vi "Main_21A.vi"() -> ()   [LabVIEW 2024]
uses:
  Cluster_Start-End Keys.ctl
  Utility/Universal Utility/TypeDefs_Utility/Cluster_Row-Column.ctl
  9e3f57c0-2ef8-4495-8287-c6a42a5fb955.vi
  Utility/Universal Utility/TypeDefs_Utility/ENUM_4 Directions U-D-L-R.ctl
  Utility/Universal Utility/TypeDefs_Utility/ENUM_8 Directions U-D-L-R.ctl
  ENUM_Numeric Keys.ctl
  ENUM_Arrow Keys.ctl
panel:
  out "concatenated string":string
  out "Array":string[](array[string])
  out "Robot 3 to 2":cluster{"Array":cluster{"Array":string[]}[]}[](array[cluster])
  out "2 to 1 Robot":cluster{"Array":string[]}[](array[cluster])
  out "counts":i32[](array[numeric])
  out "Number":i32[](array[numeric])
  in  "Select Data":enum32{"Example", "Puzzle"}(tab)
  in  "Example":string="029A\n980A\n179A\n456A\n379A"
  in  "Puzzle":string="129A\n974A\n805A\n671A\n386A"
  out "Answer":u32
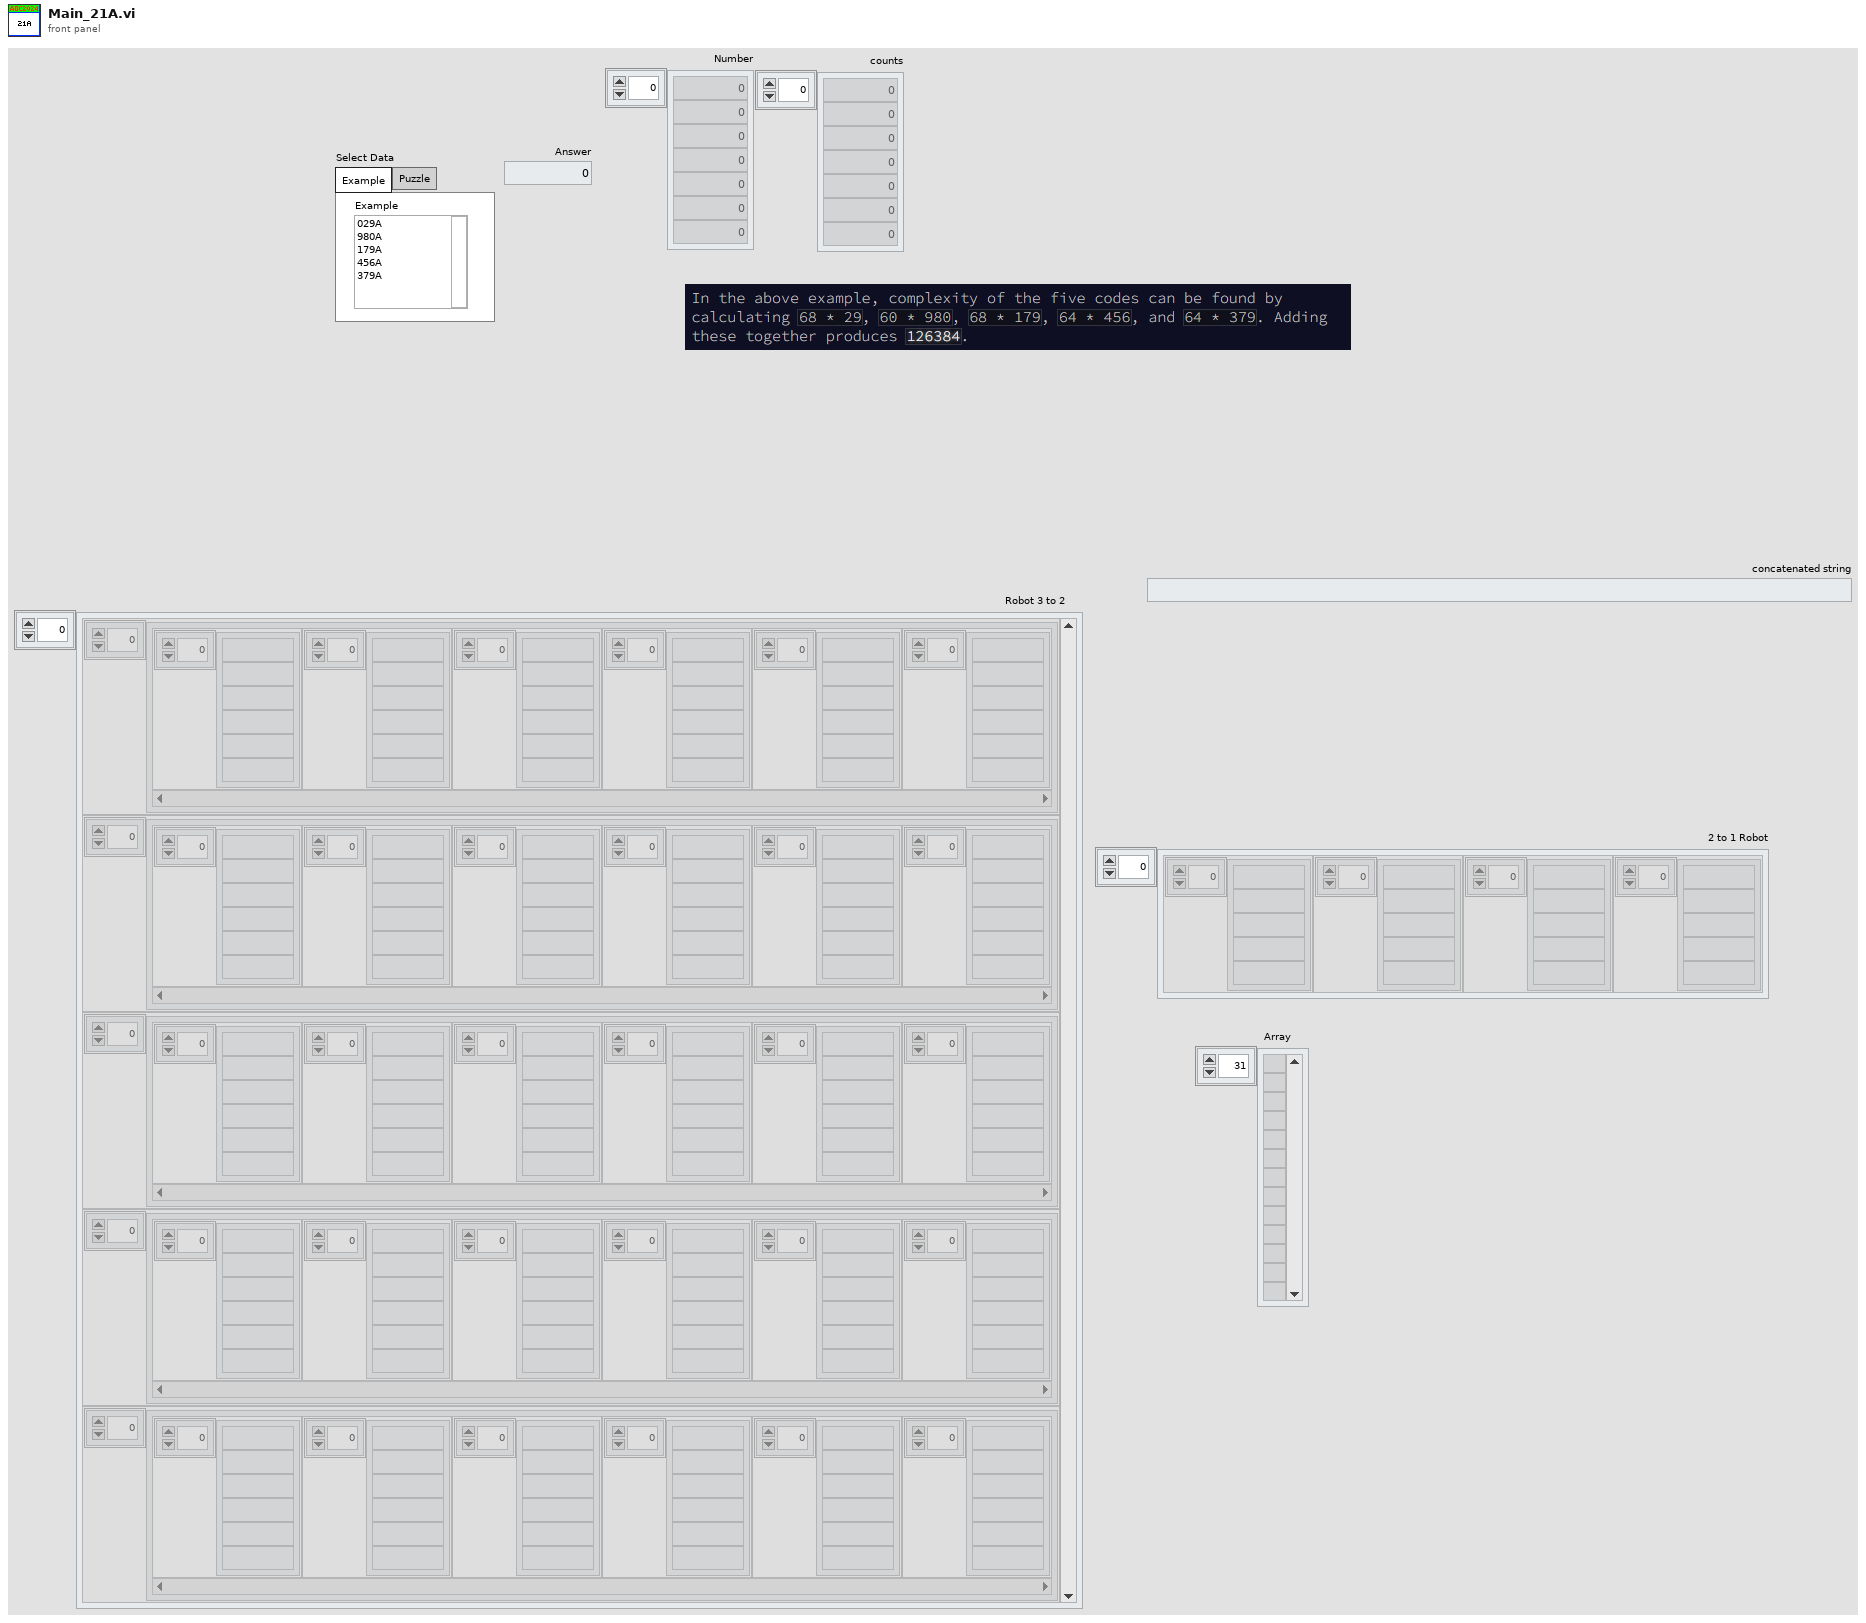
[diagram p1: front panel]
types:
  T1 = typedef "ENUM_Arrow Keys.ctl" = enum16{"#; 0,0", "^; 0,1", "A; 0,2", "<; 1,0", "v; 1,1", ">; 1,2"}
  T2 = typedef "ENUM_Numeric Keys.ctl" = enum16{"0; 3,1", "1; 2,0", "2; 2,1", "3; 2,2", "4; 1,0", "5; 1,1", "6; 1,2", "7; 0,0", "8; 0,1", "9; 0,2", "A; 3,2", "#; 3,0"}
  T3 = typedef "ENUM_8 Directions U-D-L-R.ctl" = enum16{"Up;-1,0", "Up-Right;-1,1", "Right;0,1", "Down-Right;1,1", "Down;1,0", "Down-Left;1,-1", "Left;0,-1", "Up-Left;-1,-1"}
  T4 = typedef "ENUM_4 Directions U-D-L-R.ctl" = enum16{"Up;-1,0", "Right;0,1", "Down;1,0", "Left;0,-1"}
  T5 = typedef "Cluster_Row-Column.ctl" = cluster{"R":i32, "C":i32}
  T6 = typedef "Cluster_Start-End Keys.ctl" = cluster{"Start":string, "End":string}
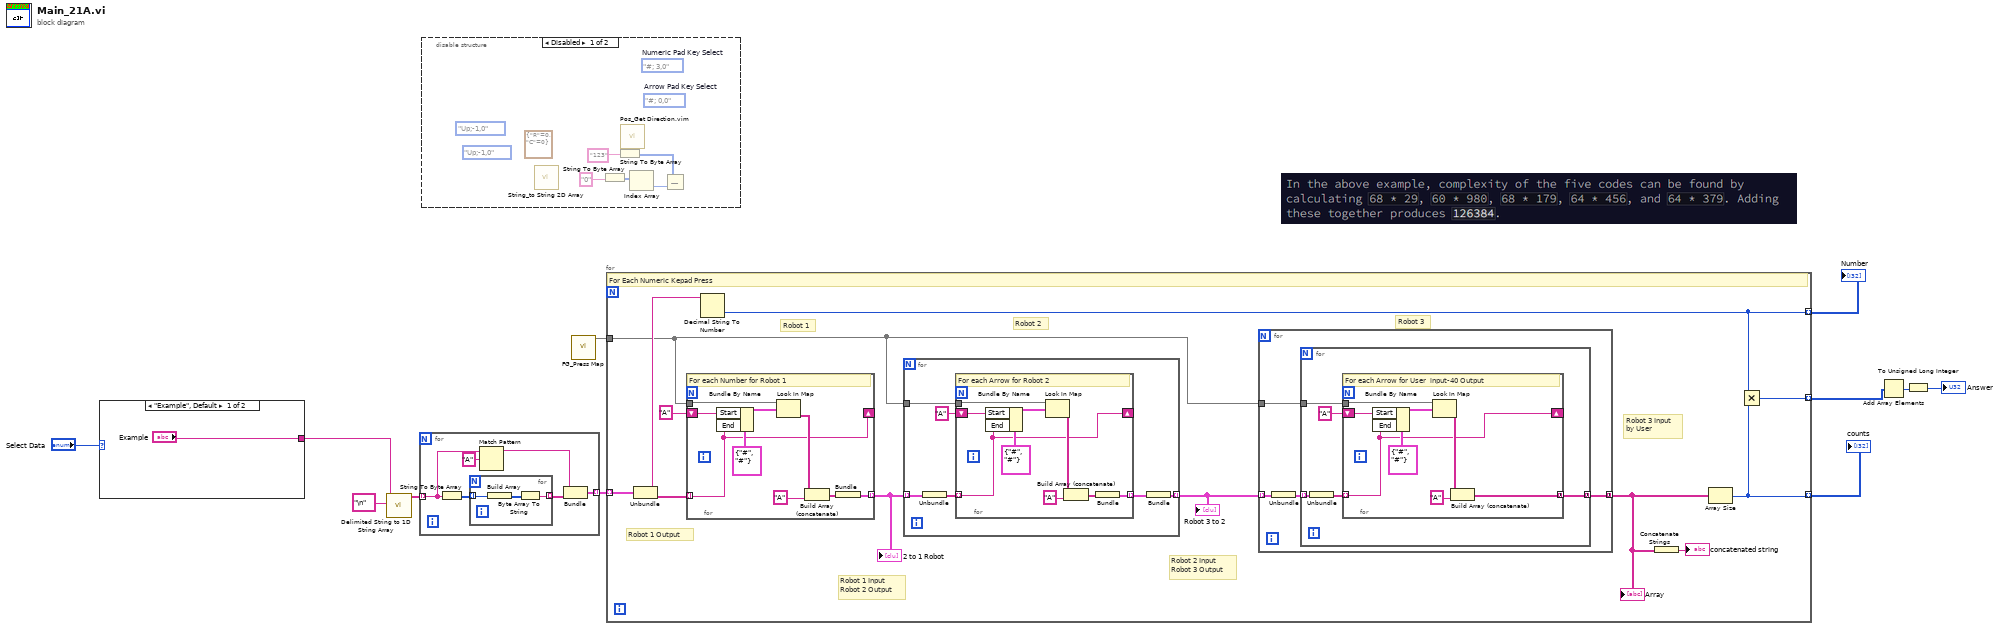
[diagram p0: block diagram]
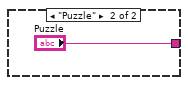
[diagram p2: hidden frame]
diagram:
  n1 = case shown="\"Example\", Default" "Select Data" {
    tunnel: ["Example" "Puzzle"] -> w7
    frame "Example", Default {
    }
    frame "Puzzle" {
    }
  }
  n2 = call <vilib>:"Delimited String to 1D String Array.vi"("delimiter"="\n" ("delimiter (Tab)"), "delimited string"=w7) -> ("string array"=w10:string[])  [unwired: 9 in]
  n3 = for {
    tunnel: w10 -> [w14] mode=indexing
    tunnel: [w17] -> w6 mode=indexing
    n4 = String To Byte Array(string=w14) -> (unsigned byte array=w19:u8[])
    n5 = for {
      tunnel: w19 -> [w22] mode=indexing
      tunnel: [w20] -> w18 mode=indexing
      n6 = Build Array(w22) -> (w21:u8[])
      n7 = Byte Array To String(unsigned byte array=w21) -> (string=w20:string)
    }
    n8 = Match Pattern(string=w14, regular expression="A") -> (before substring=w15:string)  [unwired: 1 in, 3 out]
    n9 = Bundle("String"=w15, w18) -> (w17:cluster{"String":string, string[]})  [unwired: 1 in]
  }
  n10 = disable-structure shown="Disabled" {
    frame Disabled {
      (unwired) ENUM_Arrow_Keys."#; 0,0"  # Arrow Pad Key Select
      (unwired) ENUM_Numeric_Keys."#; 3,0"  # Numeric Pad Key Select
      (unwired) ENUM_8_Directions_U-D-L-R."Up;-1,0" ("Direction 8")
      (unwired) ENUM_4_Directions_U-D-L-R."Up;-1,0" ("Direction")
      (unwired) T5 {"R"=0, "C"=0} ("Position")
      n11 = call "String_to String 2D Array.vi"() -> ()  [unwired: 11 in, 1 out]
      n12 = String To Byte Array(string="0") -> (unsigned byte array=w25:u8[])
      n13 = String To Byte Array(string="123") -> (unsigned byte array=w23:u8[])
      n14 = call "Pos_Get Direction.vim"() -> ()  [unwired: 11 in, 1 out]
      n15 = Index Array(array=w25) -> (element=w24:u8)  [unwired: 1 in]
      n16 = Subtract(x=w23, y=w24) -> ()  [unwired: 1 out]
    }
    frame Enabled {
    }
  }
  n17 = call "FG_Press Map.vi"() -> ("Press Table"=w5:map{T6, string[]})  [unwired: 11 in]
  n18 = for {
    tunnel: w6 -> [w39] mode=indexing
    tunnel: [w31] -> w4 mode=indexing
    tunnel: w5 -> [w34]
    tunnel: [w32] -> w3 mode=indexing
    tunnel: [w30] -> w1 mode=indexing
    # "Robot 3 Input\nby User"
    # "Robot 2 Input\nRobot 3 Output"
    # "Robot 1 Output"
    # "Robot 3"
    # "Robot 2"
    # "Robot 1"
    # "Robot 1 Input\nRobot 2 Output"
    # "For Each Numeric Kepad Press"
    n19 = Unbundle(w39) -> ("String"=w38:string, w37:string[])
    n20 = for {
      tunnel: w37 -> [w73] mode=indexing
      tunnel: w34 -> [w74]
      tunnel: [w72] -> w35 mode=indexing
      shift-right: [w73] -> _
      shift-left: "A" ("regular expression") -> [w79]
      # "For each Number for Robot 1"
      n21 = Bundle By Name(cluster=T6 {"Start"="#", "End"="#"} ("Start End Keys"), "Start"=w79, "End"=w73) -> (w78:T6)
      n22 = Look In Map(map=w74, key=w78) -> (value=w77:string[])  [unwired: 1 in, 1 out]
      n23 = Build Array (concatenate)(w77, "A" ("regular expression")) -> (w75:string[])
      n24 = Bundle(w75) -> (w72:cluster{string[]})  [unwired: 1 in]
    }
    "2 to 1 Robot" <- w35
    n25 = Decimal String To Number(string=w38) -> (number=w31:i32)  [unwired: 2 in, 1 out]
    n26 = for {
      tunnel: w35 -> [w62] mode=indexing
      tunnel: w34 -> [w60]
      tunnel: [w58] -> w33 mode=indexing
      n27 = Unbundle(w62) -> (w59:string[])
      n28 = for {
        tunnel: w59 -> [w64] mode=indexing
        tunnel: w60 -> [w65]
        tunnel: [w63] -> w57 mode=indexing
        shift-right: [w64] -> _
        shift-left: "A" ("regular expression") -> [w70]
        # "For each Arrow for Robot 2"
        n29 = Bundle By Name(cluster=T6 {"Start"="#", "End"="#"} ("Start End Keys"), "Start"=w70, "End"=w64) -> (w69:T6)
        n30 = Look In Map(map=w65, key=w69) -> (value=w68:string[])  [unwired: 1 in, 1 out]
        n31 = Build Array (concatenate)(w68, "A" ("regular expression")) -> (w66:string[])
        n32 = Bundle(w66) -> (w63:cluster{string[]})  [unwired: 1 in]
      }
      n33 = Bundle(w57) -> (w58:cluster{cluster{string[]}[]})  [unwired: 1 in]
    }
    "Robot 3 to 2" <- w33
    n34 = for {
      tunnel: w34 -> [w43]
      tunnel: w33 -> [w42] mode=indexing
      tunnel: [w41] -> w29 mode=concatenating
      n35 = Unbundle(w42) -> (w40:cluster{string[]}[])
      n36 = for {
        tunnel: w43 -> [w48]
        tunnel: w40 -> [w46] mode=indexing
        tunnel: [w45] -> w41 mode=concatenating
        n37 = Unbundle(w46) -> (w44:string[])
        n38 = for {
          tunnel: w44 -> [w49] mode=indexing
          tunnel: w48 -> [w50]
          tunnel: [w51] -> w45 mode=concatenating
          shift-right: [w49] -> _
          shift-left: "A" ("regular expression") -> [w55]
          # "For each Arrow for User  input-40 Output"
          n39 = Bundle By Name(cluster=T6 {"Start"="#", "End"="#"} ("Start End Keys"), "Start"=w55, "End"=w49) -> (w54:T6)
          n40 = Look In Map(map=w50, key=w54) -> (value=w53:string[])  [unwired: 1 in, 1 out]
          n41 = Build Array (concatenate)(w53, "A" ("regular expression")) -> (w51:string[])
        }
      }
    }
    "Array" <- w29
    n42 = Concatenate Strings(w29) -> (→"concatenated string":string)
    n43 = Array Size(array=w29) -> (size(s)=w32:i32)
    n44 = Multiply(x=w31, y=w32) -> (x*y=w30:i32)
  }
  "Number" <- w4
  "counts" <- w3
  n45 = Add Array Elements(numeric array=w1) -> (sum=w2:i32)
  n46 = To Unsigned Long Integer(number=w2) -> (unsigned 32bit integer=→"Answer":u32)
